vi "DeSerializeInputs.vi"(0 "object in":refnum<class "JSONJDP.lvclass">, 2 "InputTypes":variant[](array[variant]), 3 "InputString":string, 5 "error in (no error)":errorcluster) -> (14 "object out":refnum<class "JSONJDP.lvclass">, 16 "Inputs":variant[](array[variant]), 19 "error out":errorcluster)   [LabVIEW 2018, in "JSONJDP.lvclass"]
uses:
  JSONJDP.lvclass
  d8773552-9569-4127-ada2-a969fe319964.vi
  <vilib>/JDP Science/JSONtext/JSON text to Variant.vi
  <vilib>/JDP Science/JSONtext/LVClass Serializer/JSONtext LVClass Serializer.lvclass
  <vilib>/JDP Science/JSONtext/JSONtext.lvlib
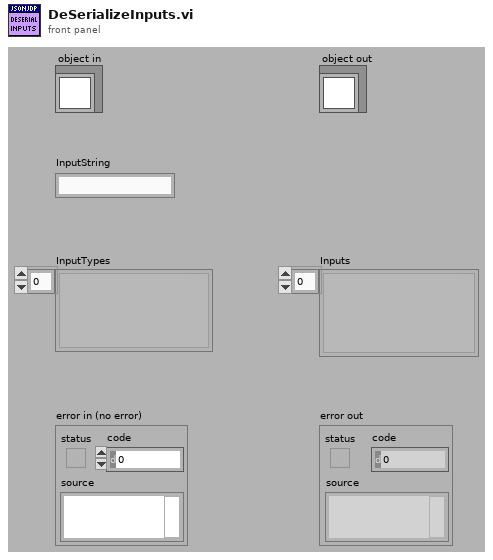
[diagram p1: front panel]
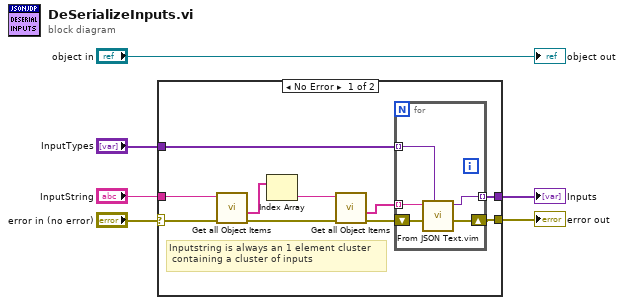
[diagram p0: block diagram]
diagram:
  n1 = case shown="No Error" "error in (no error)" {
    selector: "error in (no error)" -> [w12 w22]
    tunnel: [w16 w22] -> w5
    tunnel: "InputString" -> [w15 _]
    tunnel: "InputTypes" -> [w14 _]
    tunnel: [w13 _] -> w1
    frame No Error {
      # "Inputstring is always an 1 element cluster\n containing a cluster of inputs"
      n2 = call <vilib>:"Get all Object Items.vi"("error in (no error)"=w12, "JSON"=w15) -> ("error out"=w10:errorcluster, "<JSON>"=w9:string[])  [unwired: 6 in, 2 out]
      n3 = Index Array(array=w9) -> (element=w11:string)  [unwired: 1 in]
      n4 = call <vilib>:"Get all Object Items.vi"("error in (no error)"=w10, "JSON"=w11) -> ("error out"=w7:errorcluster, "<JSON>"=w8:string[])  [unwired: 6 in, 2 out]
      n5 = for {
        tunnel: w8 -> [w21] mode=indexing
        shift-right: [w20] -> w16
        shift-left: w7 -> [w19]
        tunnel: w14 -> [w18] mode=indexing
        tunnel: [w17] -> w13 mode=indexing
        n6 = call "From JSON Text.vim"("Data Type and Default Value"=w18, "error in (no error)"=w19, "JSON"=w21) -> ("error out"=w20:errorcluster, "Data out"=w17:variant)  [unwired: 7 in]
      }
    }
    frame Error {
    }
  }
  "error out" <- w5
  "Inputs" <- w1
  "object out" <- "object in"
